vi "GetSTL_after307.vi"(8 "error in (no error)":errorcluster, 10 "Comm in":T1, 11 "Device in":T2) -> (0 "error out":errorcluster, 1 "error":i32, 2 "Comm out":T1, 3 "Device Out":T2)   [LabVIEW 2019]
uses:
  <userlib>/Onshape/_SubVI/Cluster.ctl
  <userlib>/IoT Devices/_subVIs/HTTPComm.ctl
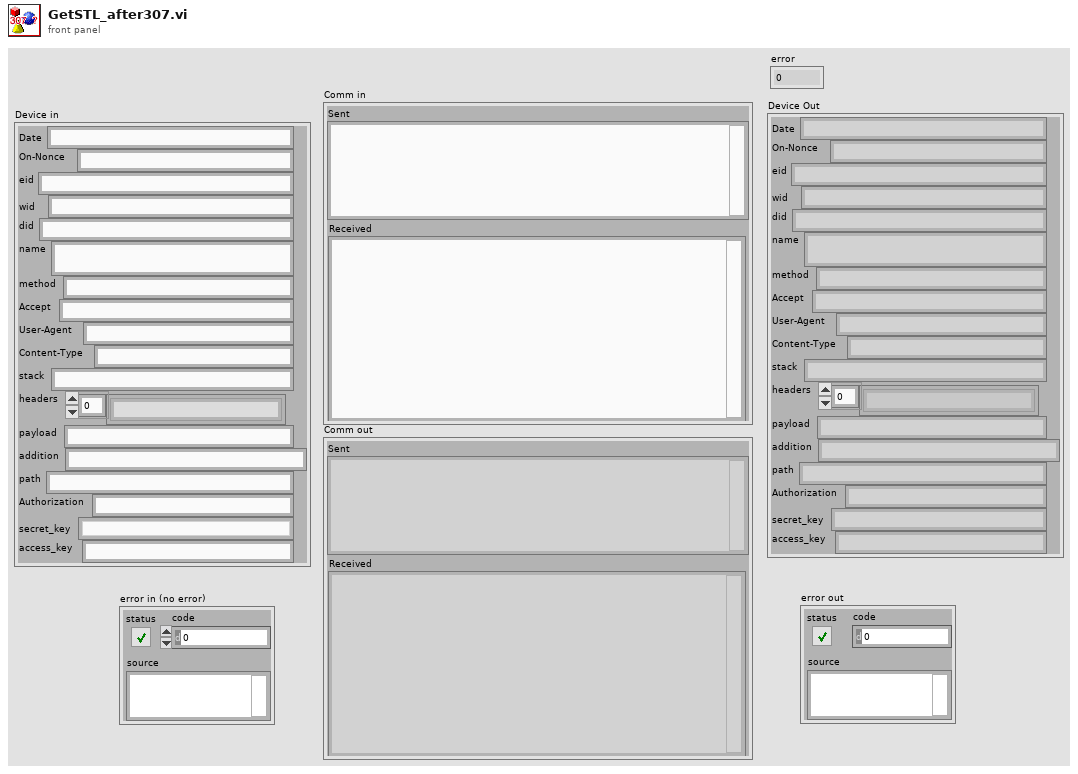
[diagram p1: front panel]
types:
  T1 = typedef "HTTPComm.ctl" = cluster{"url":string, "sent headers":string, "sent body":string, "headers":string, "body":string, "Sent":string, "Received":string}
  T2 = typedef "Cluster.ctl" = cluster{"Date":string, "On-Nonce":string, "eid":string, "wid":string, "did":string, "name":string, "method":string, "Accept":string, "User-Agent":string, "Content-Type":string, "stack":string, "headers":string[], "payload":string, "addition":string, "path":string, "Authorization":string, "secret_key":string, "access_key":string}
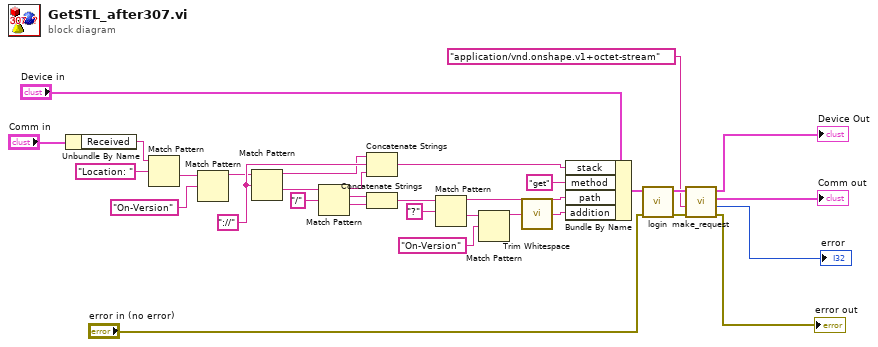
[diagram p0: block diagram]
diagram:
  w13 = "://" ("regular expression")
  n1 = Unbundle By Name("Comm in") -> ("Received"=w5:string)
  n2 = Match Pattern(string=w5, regular expression="Location: ") -> (after substring=w7:string)  [unwired: 1 in, 3 out]
  n3 = Match Pattern(string=w7, regular expression="On-Version") -> (before substring=w9:string)  [unwired: 1 in, 3 out]
  n4 = Match Pattern(string=w9, regular expression=w13) -> (before substring=w12:string, after substring=w11:string)  [unwired: 1 in, 2 out]
  n5 = Match Pattern(string=w11, regular expression="/") -> (before substring=w14:string, match substring=w19:string, after substring=w20:string)  [unwired: 1 in, 1 out]
  n6 = Concatenate Strings(w12, w13, w14) -> (w22:string)
  n7 = Concatenate Strings(w19, w20) -> (w21:string)
  n8 = Match Pattern(string=w21, regular expression="?") -> (before substring=w17:string, after substring=w29:string)  [unwired: 1 in, 2 out]
  n9 = Match Pattern(string=w29, regular expression="On-Version") -> (before substring=w31:string)  [unwired: 1 in, 3 out]
  n10 = call <vilib>:"Trim Whitespace.vi"("string"=w31) -> ("trimmed string"=w32:string)  [unwired: 1 in]
  n11 = Bundle By Name(cluster="Device in", "stack"=w22, "method"="get", "path"=w17, "addition"=w32) -> (w27:T2)
  n12 = call <userlib>:"login.vi"("error in"="error in (no error)", "Device In"=w27) -> ("error out"=w2:errorcluster, "Device Out"=w28:T2)  [unwired: 8 in]
  n13 = call <userlib>:"make_request.vi"("Error in"=w2, "Accept"="application/vnd.onshape.v1+octet-stream", "Device In"=w28) -> ("error out"=→"error out":errorcluster, "error"=→"error":i32, "Comm"=→"Comm out":T1, "Device Out"=→"Device Out":T2)  [unwired: 4 in, 1 out]
